vi "Send Receive SPTI Command.vi"(6 "read/write":enum16{"Read", "Write"}(ring), 7 "Data to be Written":u8[](array[numeric]), 8 "error in (no error)":errorcluster, 9 "Expected Nr Response Bytes":i32=36, 10 "Valid CDB bytes":u8=6, 11 "Command Data Block":u8[](array[numeric])=[18, 0, 0, 0, 36, 0, 0, 0, 0, 0, 0, 0, 0, 0, 0, 0] format="%02x") -> (0 "error out":errorcluster, 3 "Received Data":u8[](array[numeric]) format="%02x")   [LabVIEW 2014]
uses:
  BasicDLL.dll
panel:
  out "Nr Bytes Received":i32
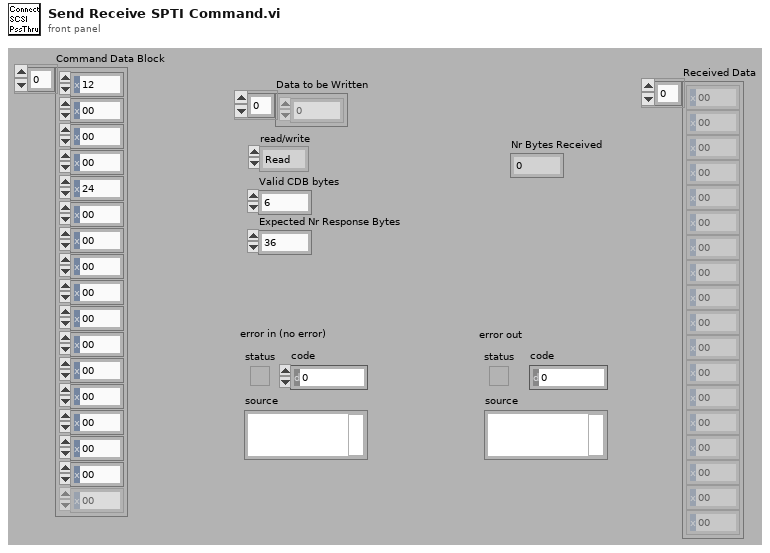
[diagram p1: front panel]
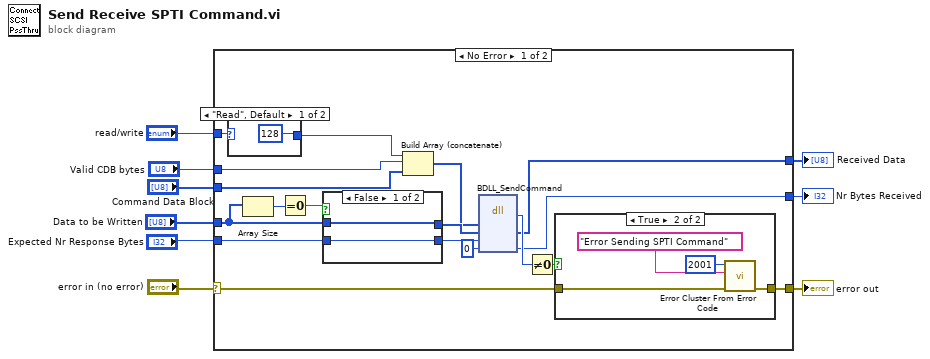
[diagram p0: block diagram]
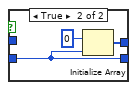
[diagram p2: hidden frame]
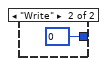
[diagram p3: hidden frame]
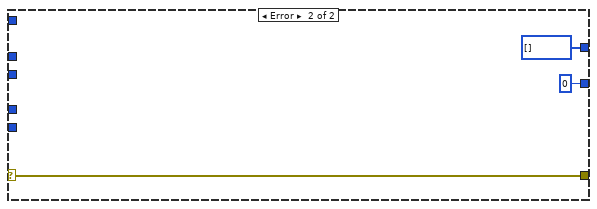
[diagram p5: hidden frame]
diagram:
  n1 = case shown="No Error" "error in (no error)" {
    selector: "error in (no error)" -> [w24 w42]
    tunnel: [w27 w42] -> w9
    tunnel: "Expected Nr Response Bytes" -> [w22 _]
    tunnel: "read/write" -> [w20 _]
    tunnel: "Valid CDB bytes" -> [w18 _]
    tunnel: "Command Data Block" -> [w17 _]
    tunnel: [w15 u8[] [] ("data_ptr")] -> w2
    tunnel: [w14 0 ("actual_received")] -> w3
    tunnel: "Data to be Written" -> [w10 _]
    frame No Error {
      n2 = case shown="\"Read\", Default" w20 {
        tunnel: [u8 128 u8 0] -> w19
        frame "Read", Default {
        }
        frame "Write" {
        }
      }
      n3 = Array Size(array=w10) -> (size(s)=w13:i32)
      n4 = Equal To 0?(x=w13) -> (x = 0?=w12:bool)
      n5 = case shown="False" w12 {
        tunnel: w22 -> [w28 w30]
        tunnel: [w29 w31] -> w21
        tunnel: [w28 w30] -> w11
        tunnel: w10 -> [w29 _]
        frame False {
        }
        frame True {
          n6 = Initialize Array(u8 0 ("element"), w30) -> (w31:u8[])
        }
      }
      n7 = Build Array (concatenate)(w19, w18, w17) -> (w16:u8[])
      n8 = dll-call lib="C:/Users/SingleCell/Desktop/Biostinger/BioStingerGUI/Gener8 Software/Low Level USB/Low Level USB/BasicDLL.dll" fn="BDLL_SendCommand"("command"=w16, "data_ptr"=w21, "num_received"=w11, "actual_received"=0) -> (w25:i32, "data_ptr"=w15:u8[], "actual_received"=w14:i32)  [unwired: 5 in, 2 out]
      n9 = Not Equal To 0?(x=w25) -> (x != 0?=w26:bool)
      n10 = case shown="True" w26 {
        tunnel: [w35 w39] -> w27
        tunnel: w24 -> [w35 w38]
        frame False {
        }
        frame True {
          n11 = call <vilib>:"Error Cluster From Error Code.vi"("error in (no error)"=w38, "error message (\"\")"="Error Sending SPTI Command" ("error message (\"\")"), "error code (0)"=2001) -> ("error out"=w39:errorcluster)  [unwired: 6 in]
        }
      }
    }
    frame Error {
    }
  }
  "error out" <- w9
  "Received Data" <- w2
  "Nr Bytes Received" <- w3
